vi "Write Integrate Configuration.vi"(8 "error in (no error)":errorcluster, 10 "Configuration":T1={"Integrate"=[], "Offset duration "=0.0095, "TDMS group name"="p"} {"Offset duration" format="%#_6ps"; "Integrate"."Duration" format="%#_6ps"; "Integrate"."Start time" format="%#_6ps"}, 11 "Integrate in":refnum<class "Integrate.lvclass">) -> (0 "error out":errorcluster, 3 "Integrate out":refnum<class "Integrate.lvclass">)   [LabVIEW 2016, in "Integrate.lvclass"]
uses:
  Integrate.lvclass
  C:/github/LabActor/Template Module/Template Module.lvclass
  Integrator Configuration.ctl
  NHMFL_Core/Libraries/Utilities/Controls/Integrate channel.ctl
  Template Module/Template Module.lvclass/Template Module.ctl
  Template Module/Write Configuration.vi
panel:
  # "Input CH"
  # "X-Factor"
  # "Output CH"
  # "Start"
  # "Duration"
  # "Fix drift"
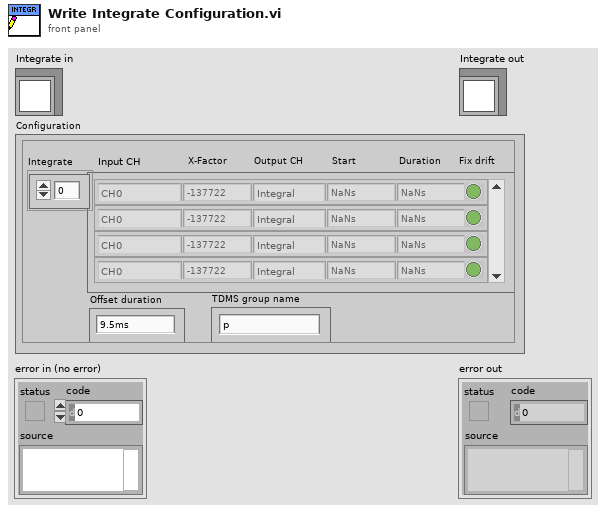
[diagram p1: front panel]
types:
  T1 = typedef "Integrator Configuration.ctl" = cluster{"Integrate":T2[], "Offset duration ":dbl, "TDMS group name":string}
  T2 = typedef "Integrate channel.ctl" = cluster{"Channel":string, "Output name":string, "Factor":dbl, "Start time":dbl, "Duration":dbl, "Fix drift":bool}
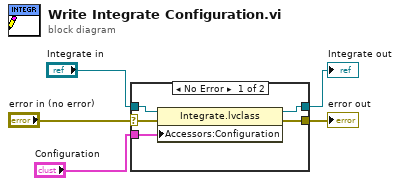
[diagram p0: block diagram]
diagram:
  n1 = case shown="No Error" "error in (no error)" {
    selector: "error in (no error)" -> [w7 w11]
    tunnel: [w6 w11] -> w4
    tunnel: [w9 w12] -> w2
    tunnel: "Integrate in" -> [w10 w12]
    tunnel: "Configuration" -> [w8 _]
    frame No Error {
      n2 = property class="Integrate.lvclass"(reference=w10, error in=w7, "Accessors:Configuration"=w8) -> (reference out=w9:refnum<class "Integrate.lvclass">, error out=w6:errorcluster)
    }
    frame Error {
    }
  }
  "error out" <- w4
  "Integrate out" <- w2
